vi "Anritsu Power Meter Control Panel (No Objects).vi"(8 "error in (no error)":errorcluster) -> (0 "error out":errorcluster)   [LabVIEW 2009]
doc: "(Dynamic) A user-level application that simulates the physical front panel of the Instrument. Provide the user with buttons to manually control features of the instrument, and provide indicators of its current state."
uses:
  Anritsu Power Meter/Public/Display control.ctl
  Anritsu Power Meter/Public/Range control watts and dBm.ctl
  Anritsu Power Meter/Public/Measuring rate control.ctl
  Anritsu Power Meter/Public/Range Status.ctl
  Anritsu Power Meter/Public/Auto Range control.ctl
  Anritsu Power Meter/Public/Averaging control.ctl
panel:
  in  "VISA Resource Name":refnum<visa-resource-name>="GPIB0::21::INSTR"
  in  "Cluster In":T6={"Averaging"=enum."On", "Units"=enum."Watt", "Measuring rate"=enum."Hold", "Unit Range"=enum."10 mW (+10 dBm)", "Calibration Factor"=-26.67, "Auto Ranging?"=enum."Off"}
  in  "Set Calibration Factor":dbl=-26.67 format="%#5_4g"
  in  "Specify Calibration Factor":bool
  in  "Auto range? 2":bool
  in  "Set Auto Range":T5
  in  "Set Averaging":T1
  out "Averaging":T1
  out "Auto Ranging?":T5
  out "In Range?":T7
  out "Power number":dbl
  out "Power":string
  in  "Set Zero":bool
  in  "Set Unit Range":T4
  in  "Set Measuring Rate":T3
  in  "Specify Range Command":bool
  in  "Set Units":T2
  out "Calibration Factor":dbl
  out "Unit Range":T4
  out "Units":T2
  in  "Query Everything":bool
  in  "Select Measurement Rate":bool
  in  "Averaging?":bool
  in  "Select Unit Display":bool
  in  "Auto range?":bool
  in  "Stop":bool
  in  "Copy actual to set":bool
  in  "Populate fields with member data":bool
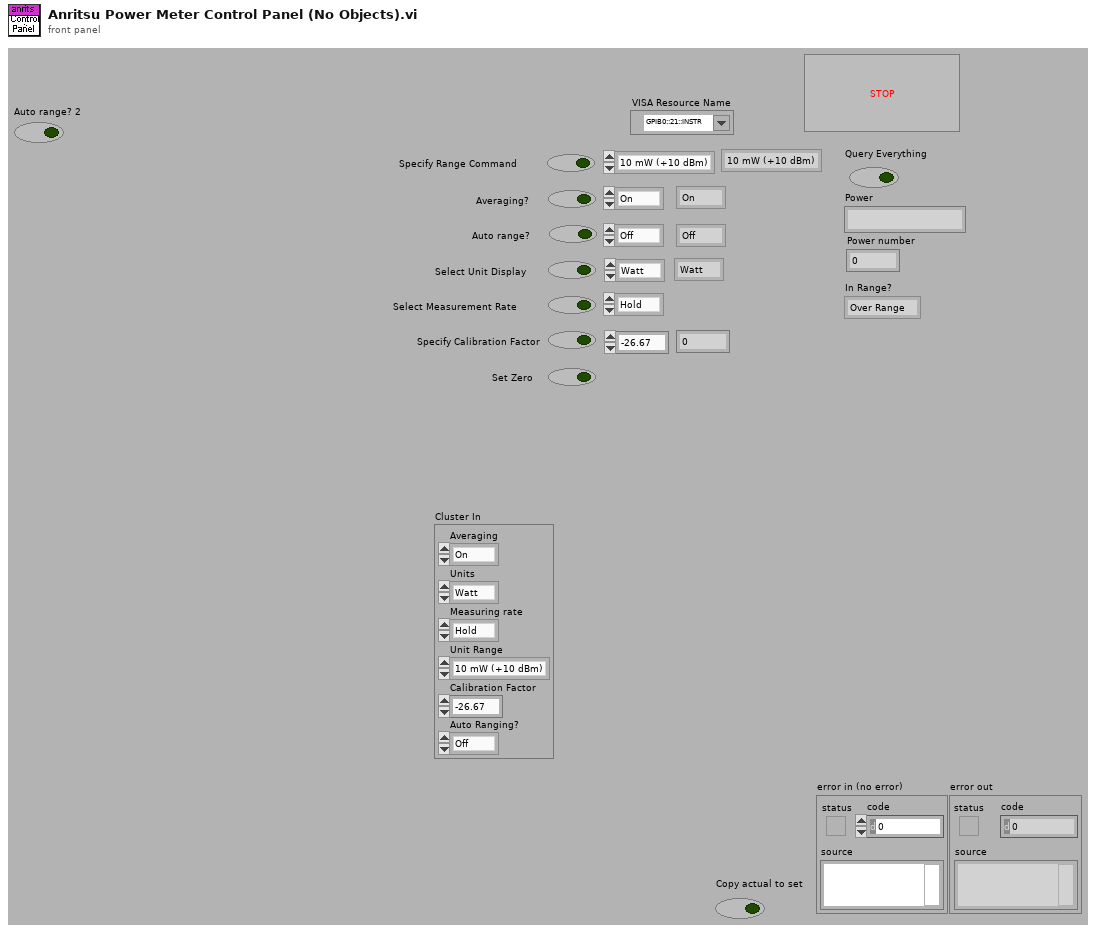
[diagram p1: front panel]
types:
  T1 = typedef "Averaging control.ctl" = enum16{"On", "Off"}
  T2 = typedef "Display control.ctl" = enum16{"Watt", "dBm", "dB (REL)"}
  T3 = typedef "Measuring rate control.ctl" = enum16{"Hold", "Free Run", "Exit Trigger"}
  T4 = typedef "Range control watts and dBm.ctl" = enum16{"10 mW (+10 dBm)", "1 mW (0 dBm)", "100 uW (-10 dBm)", "10 uW (-20 dBm)", "1 uW (-30 dBm)", "100 nW (-40 dBm)", "10 nW (-50 dBm)", "1 nW (-60 dBm)", "100 pW (-70 dBm)", "10 pW (-80 dBm)"}
  T5 = typedef "Auto Range control.ctl" = enum16{"Off", "On"}
  T6 = cluster{"Averaging":T1, "Units":T2, "Measuring rate":T3, "Unit Range":T4, "Calibration Factor":dbl, "Auto Ranging?":T5}
  T7 = typedef "Range Status.ctl" = enum16{"Over Range", "Under Range", "In Range"}
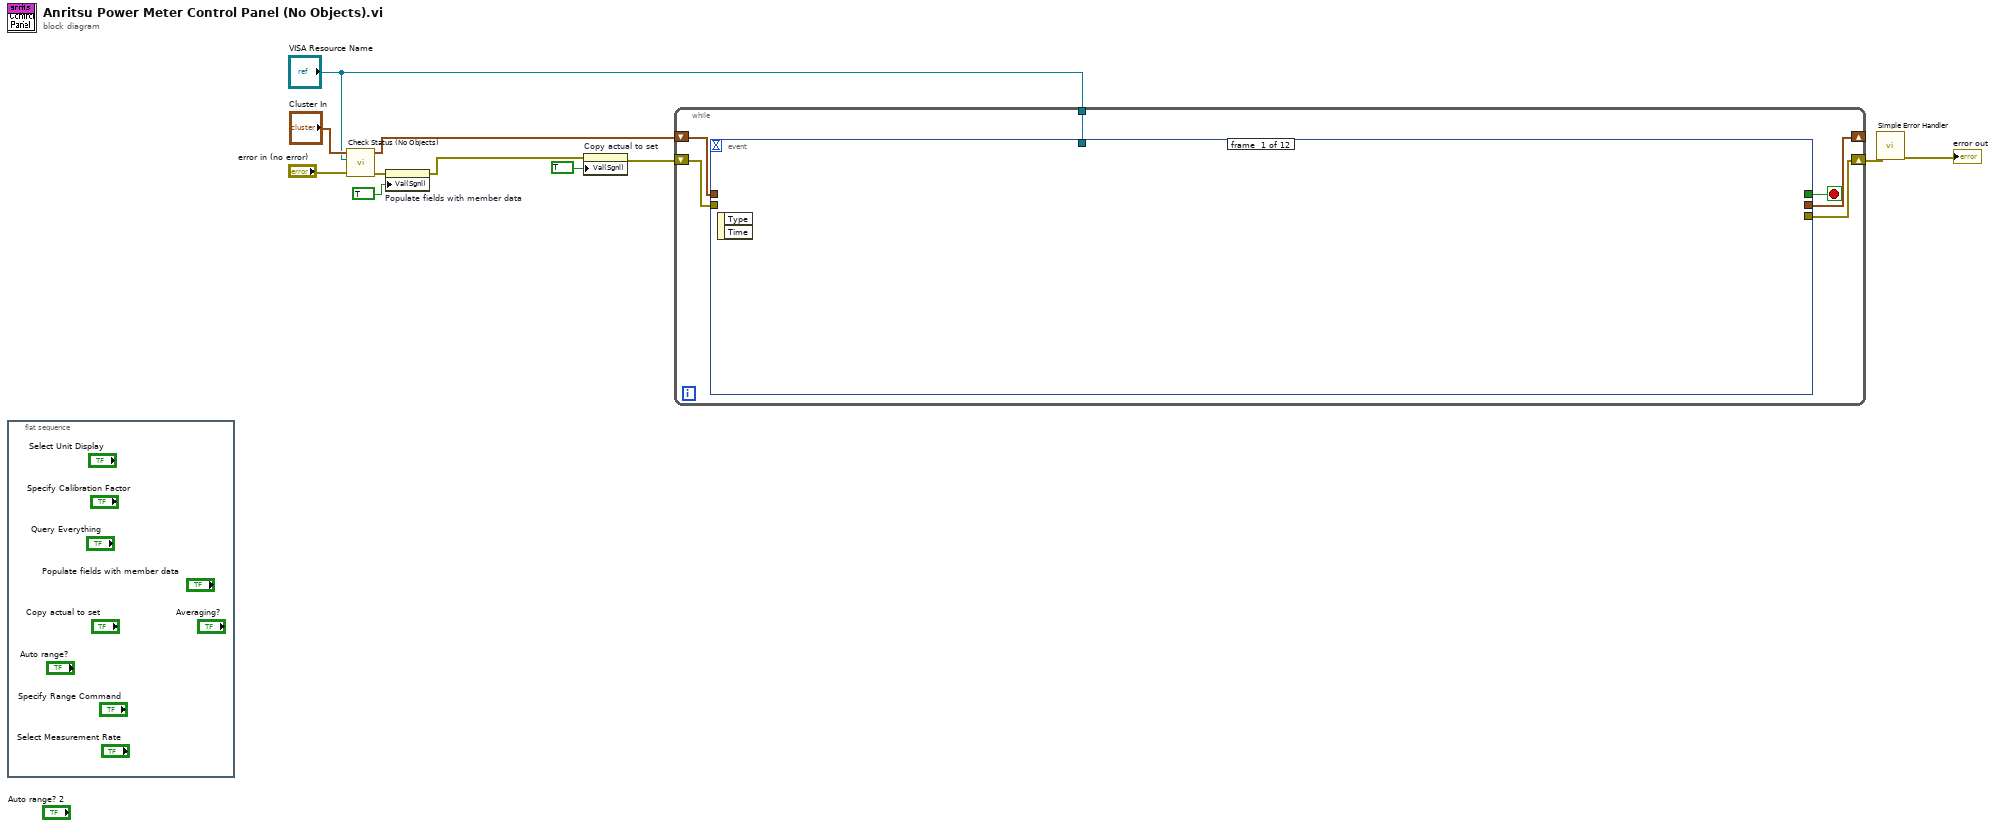
[diagram p0: block diagram]
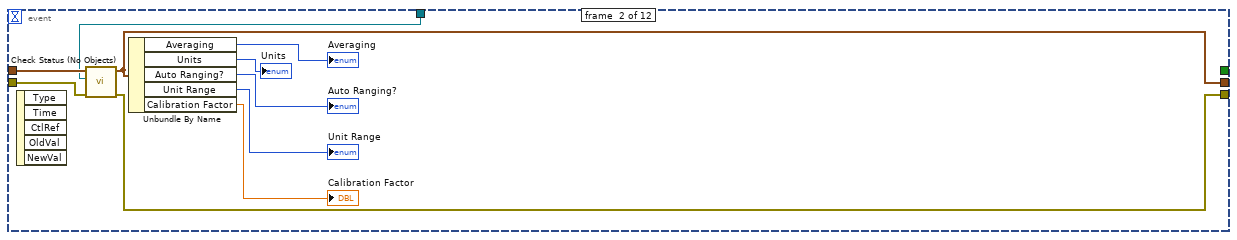
[diagram p2: hidden frame]
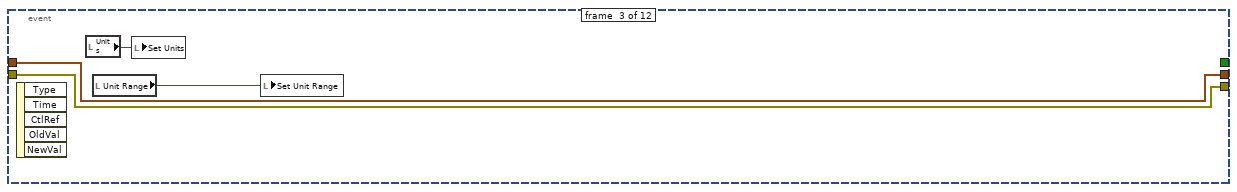
[diagram p3: hidden frame]
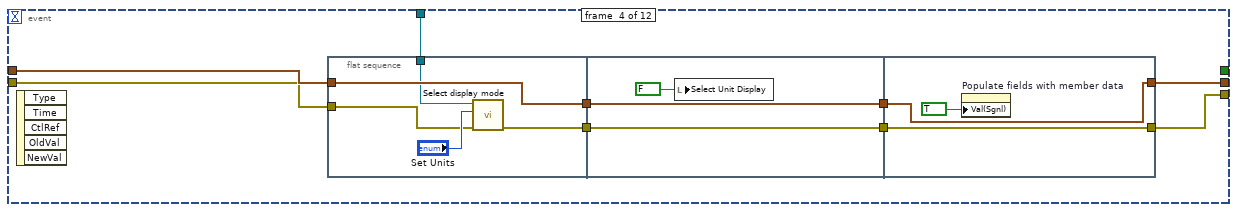
[diagram p4: hidden frame]
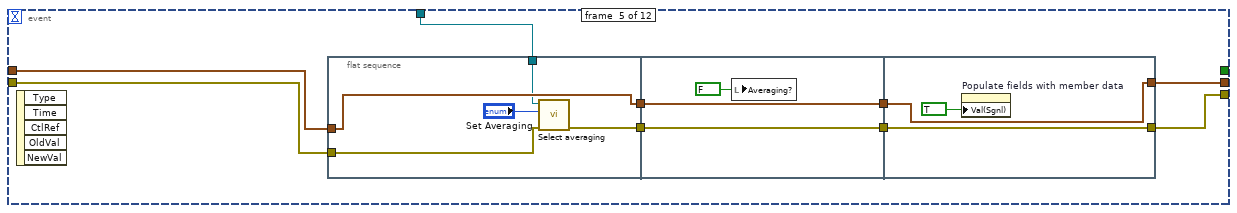
[diagram p5: hidden frame]
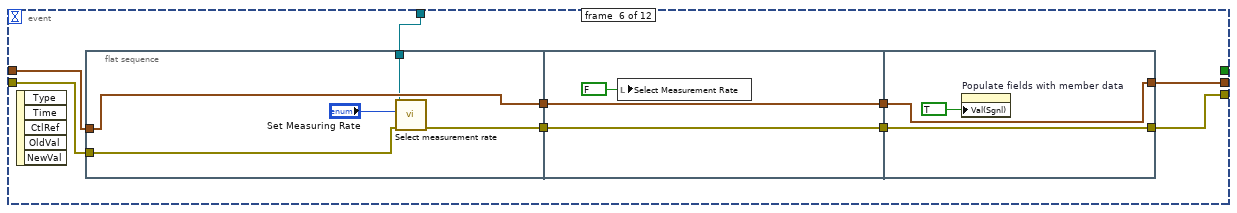
[diagram p6: hidden frame]
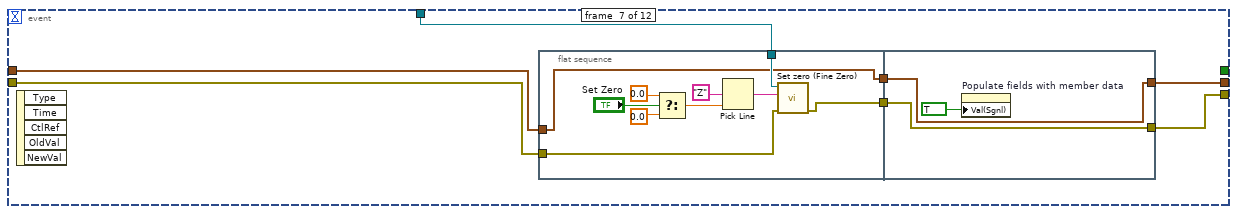
[diagram p7: hidden frame]
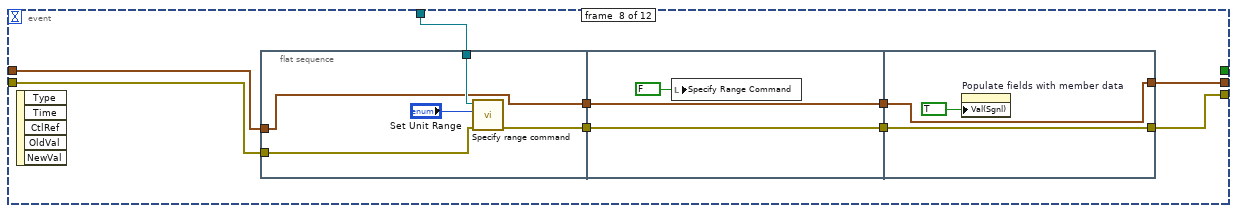
[diagram p8: hidden frame]
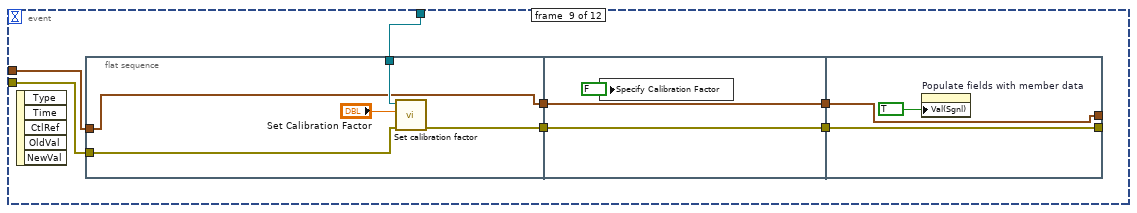
[diagram p9: hidden frame]
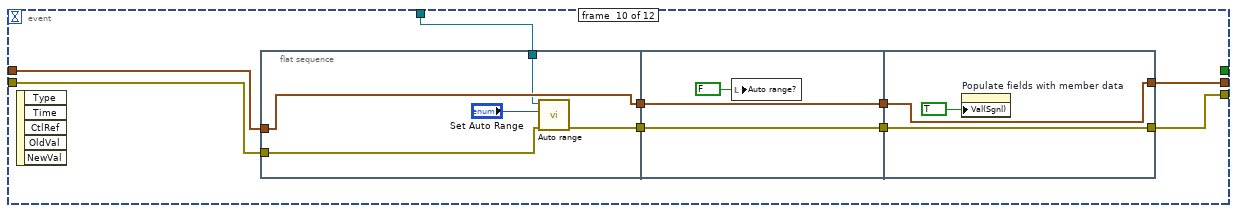
[diagram p10: hidden frame]
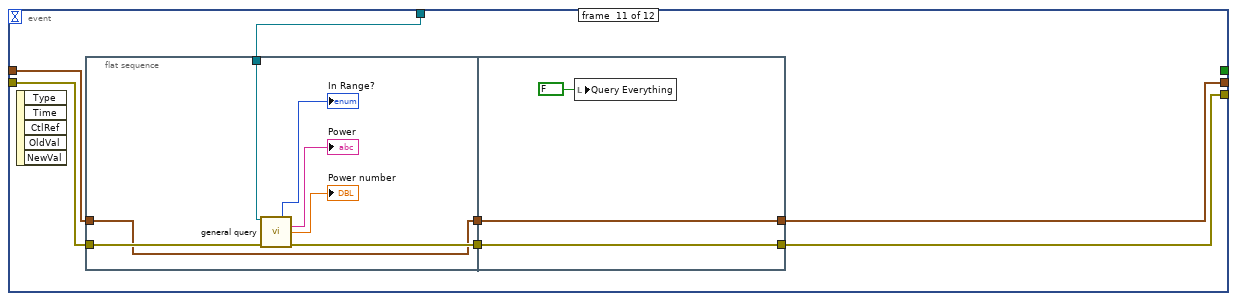
[diagram p11: hidden frame]
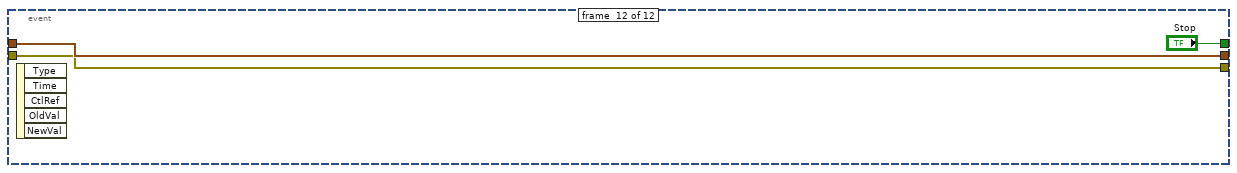
[diagram p12: hidden frame]
diagram:
  n1 = flat-sequence {
    frame #0 {
    }
  }
  n2 = call "Check Status (No Objects).vi"("error in (no error)"="error in (no error)", "VISA Resource Name"="VISA Resource Name", "Cluster In"="Cluster In") -> ("error out"=w10:errorcluster, "Cluster Out"=w8:T6)  [unwired: 5 in, 2 out]
  n3 = property on="Populate fields with member data" class="Bool (strict)"(error in=w10, "Val(Sgnl)"=TRUE ("Value (Signaling)")) -> (error out=w11:errorcluster)  [unwired: 1 in, 1 out]
  n4 = property on="Copy actual to set" class="Bool (strict)"(error in=w11, "Val(Sgnl)"=TRUE ("Value (Signaling)")) -> (error out=w9:errorcluster)  [unwired: 1 in, 1 out]
  n5 = while {
    shift-right: [w15] -> _
    shift-left: w8 -> [w16]
    shift-right: [w14] -> w5
    shift-left: w9 -> [w17]
    tunnel: "VISA Resource Name" -> [w12]
    stop <- w13 stop-if-true
    n6 = event shown="[9] \"Auto range?\": Value Change" {
      selector: _ -> [_ _ _ _ _ _ _ _ _ _ _ _]
      dyn-events: _ -> [_ _ _ _ _ _ _ _ _ _ _ _]
      timeout: _ -> [_ _ _ _ _ _ _ _ _ _ _ _]
      tunnel: w17 -> [_ w23 w28 w39 w59 w79 w97 w117 w133 w157 w176 w188]
      tunnel: w16 -> [_ w24 w29 w40 w60 w80 w98 w118 w134 w158 w175 w189]
      tunnel: [_ w22 w29 w34 w58 w78 w96 w113 _ w156 w172 w189] -> w15
      tunnel: [_ w21 w28 w33 w57 w77 w95 w114 _ w155 w171 w188] -> w14
      tunnel: [_ _ _ _ _ _ _ _ _ _ _ "Stop"] -> w13
      tunnel: w12 -> [_ w18 _ w32 w52 w72 w92 w112 w132 w150 w170 _]
      event #0 {
        n7 = event-data() -> ()  [unwired: 1 in, 2 out]
      }
      event #1 {
        n8 = event-data() -> ()  [unwired: 1 in, 5 out]
        n9 = call "Check Status (No Objects).vi"("error in (no error)"=w23, "VISA Resource Name"=w18, "Cluster In"=w24) -> ("error out"=w21:errorcluster, "Cluster Out"=w22:T6)  [unwired: 5 in, 2 out]
        n10 = Unbundle By Name(w22) -> ("Averaging"=→"Averaging":T1, "Units"=→"Units":T2, "Auto Ranging?"=→"Auto Ranging?":T5, "Unit Range"=→"Unit Range":T4, "Calibration Factor"=→"Calibration Factor":dbl)
      }
      event #2 {
        n11 = event-data() -> ()  [unwired: 1 in, 5 out]
        n12 = local read "Units"() -> (w31:T2)
        n13 = local read "Unit Range"() -> (w30:T4)
        n14 = local write "Set Units"(w31) -> ()
        n15 = local write "Set Unit Range"(w30) -> ()
      }
      event #3 {
        n16 = event-data() -> ()  [unwired: 1 in, 5 out]
        n17 = flat-sequence {
          tunnel: w40 -> [w44]
          tunnel: w39 -> [w43]
          tunnel: [w44] -> w38
          tunnel: [w41] -> w37
          tunnel: w32 -> [w42]
          tunnel: w38 -> [w47]
          tunnel: w37 -> [w46]
          tunnel: [w47] -> w36
          tunnel: [w46] -> w35
          tunnel: w36 -> [w50]
          tunnel: w35 -> [w49]
          tunnel: [w50] -> w34
          tunnel: [w49] -> w33
          frame #0 {
            n18 = call "Select display mode.vi"("error in (no error)"=w43, "Display"="Set Units", "VISA resource name"=w42) -> ("error out"=w41:errorcluster)  [unwired: 7 in, 1 out]
          }
          frame #1 {
            n19 = local write "Select Unit Display"(FALSE) -> ()
          }
          frame #2 {
            n20 = property on="Populate fields with member data" class="Bool (strict)"("Val(Sgnl)"=TRUE ("Value (Signaling)")) -> ()  [unwired: 2 in, 2 out]
          }
        }
      }
      event #4 {
        n21 = event-data() -> ()  [unwired: 1 in, 5 out]
        n22 = flat-sequence {
          tunnel: w60 -> [w63]
          tunnel: w59 -> [w61]
          tunnel: [w63] -> w56
          tunnel: [w64] -> w54
          tunnel: w52 -> [w62]
          tunnel: w56 -> [w68]
          tunnel: [w68] -> w55
          tunnel: w54 -> [w67]
          tunnel: [w67] -> w53
          tunnel: w55 -> [w70]
          tunnel: w53 -> [w69]
          tunnel: [w70] -> w58
          tunnel: [w69] -> w57
          frame #0 {
            n23 = call "Select averaging.vi"("error in (no error)"=w61, "Averaging"="Set Averaging", "VISA resource name"=w62) -> ("error out"=w64:errorcluster)  [unwired: 7 in, 1 out]
          }
          frame #1 {
            n24 = local write "Averaging?"(FALSE) -> ()
          }
          frame #2 {
            n25 = property on="Populate fields with member data" class="Bool (strict)"("Val(Sgnl)"=TRUE ("Value (Signaling)")) -> ()  [unwired: 2 in, 2 out]
          }
        }
      }
      event #5 {
        n26 = event-data() -> ()  [unwired: 1 in, 5 out]
        n27 = flat-sequence {
          tunnel: w80 -> [w83]
          tunnel: w79 -> [w82]
          tunnel: [w83] -> w76
          tunnel: [w84] -> w74
          tunnel: w72 -> [w81]
          tunnel: w76 -> [w88]
          tunnel: [w88] -> w75
          tunnel: w74 -> [w87]
          tunnel: [w87] -> w73
          tunnel: w75 -> [w90]
          tunnel: w73 -> [w89]
          tunnel: [w90] -> w78
          tunnel: [w89] -> w77
          frame #0 {
            n28 = call "Select measurement rate.vi"("error in (no error)"=w82, "Rate"="Set Measuring Rate", "VISA resource name"=w81) -> ("error out"=w84:errorcluster)  [unwired: 7 in, 1 out]
          }
          frame #1 {
            n29 = local write "Select Measurement Rate"(FALSE) -> ()
          }
          frame #2 {
            n30 = property on="Populate fields with member data" class="Bool (strict)"("Val(Sgnl)"=TRUE ("Value (Signaling)")) -> ()  [unwired: 2 in, 2 out]
          }
        }
      }
      event #6 {
        n31 = event-data() -> ()  [unwired: 1 in, 5 out]
        n32 = flat-sequence {
          tunnel: w97 -> [w100]
          tunnel: w98 -> [w99]
          tunnel: [w99] -> w94
          tunnel: [w102] -> w93
          tunnel: w92 -> [w101]
          tunnel: w94 -> [w110]
          tunnel: w93 -> [w109]
          tunnel: [w110] -> w96
          tunnel: [w109] -> w95
          frame #0 {
            n33 = Select(t=0.0, s="Set Zero", f=0.0) -> (s? t:f=w106:dbl)
            n34 = Pick Line(multi-line string="Z", line index=w106) -> (output string=w104:string)  [unwired: 1 in]
            n35 = call "Set zero (Fine Zero).vi"("error in (no error)"=w100, "Code"=w104, "VISA resource name"=w101) -> ("error out"=w102:errorcluster)  [unwired: 7 in, 1 out]
          }
          frame #1 {
            n36 = property on="Populate fields with member data" class="Bool (strict)"("Val(Sgnl)"=TRUE ("Value (Signaling)")) -> ()  [unwired: 2 in, 2 out]
          }
        }
      }
      event #7 {
        n37 = event-data() -> ()  [unwired: 1 in, 5 out]
        n38 = flat-sequence {
          tunnel: [w123] -> w120
          tunnel: [w122] -> w119
          tunnel: w118 -> [w123]
          tunnel: w117 -> [w121]
          tunnel: w112 -> [w124]
          tunnel: w120 -> [w127]
          tunnel: w119 -> [w126]
          tunnel: [w127] -> w116
          tunnel: [w126] -> w115
          tunnel: w116 -> [w130]
          tunnel: w115 -> [w129]
          tunnel: [w130] -> w113
          tunnel: [w129] -> w114
          frame #0 {
            n39 = call "Specify range command.vi"("error in (no error)"=w121, "Range"="Set Unit Range", "VISA resource name"=w124) -> ("error out"=w122:errorcluster)  [unwired: 7 in, 1 out]
          }
          frame #1 {
            n40 = local write "Specify Range Command"(FALSE) -> ()
          }
          frame #2 {
            n41 = property on="Populate fields with member data" class="Bool (strict)"("Val(Sgnl)"=TRUE ("Value (Signaling)")) -> ()  [unwired: 2 in, 2 out]
          }
        }
      }
      event #8 {
        n42 = event-data() -> ()  [unwired: 1 in, 5 out]
        n43 = flat-sequence {
          tunnel: [w139] -> w138
          tunnel: [w142] -> w137
          tunnel: w134 -> [w139]
          tunnel: w133 -> [w140]
          tunnel: w132 -> [w141]
          tunnel: w138 -> [w146]
          tunnel: [w146] -> w136
          tunnel: w137 -> [w145]
          tunnel: [w145] -> w135
          tunnel: w136 -> [w149]
          tunnel: w135 -> [w148]
          tunnel: [w149] -> _
          tunnel: [w148] -> _
          frame #0 {
            n44 = call "Set calibration factor.vi"("error in (no error)"=w140, "Calibration Factor"="Set Calibration Factor", "VISA resource name"=w141) -> ("error out"=w142:errorcluster)  [unwired: 7 in, 1 out]
          }
          frame #1 {
            n45 = local write "Specify Calibration Factor"(FALSE) -> ()
          }
          frame #2 {
            n46 = property on="Populate fields with member data" class="Bool (strict)"("Val(Sgnl)"=TRUE ("Value (Signaling)")) -> ()  [unwired: 2 in, 2 out]
          }
        }
      }
      event #9 {
        n47 = event-data() -> ()  [unwired: 1 in, 5 out]
        n48 = flat-sequence {
          tunnel: [w162] -> w153
          tunnel: w158 -> [w161]
          tunnel: w157 -> [w159]
          tunnel: [w161] -> w151
          tunnel: w150 -> [w160]
          tunnel: [w166] -> w154
          tunnel: w153 -> [w165]
          tunnel: [w165] -> w152
          tunnel: w151 -> [w166]
          tunnel: w154 -> [w169]
          tunnel: w152 -> [w168]
          tunnel: [w169] -> w156
          tunnel: [w168] -> w155
          frame #0 {
            n49 = call "Auto range.vi"("error in (no error)"=w159, "Auto Ranging?"="Set Auto Range", "VISA resource name"=w160) -> ("error out"=w162:errorcluster)  [unwired: 7 in, 1 out]
          }
          frame #1 {
            n50 = local write "Auto range?"(FALSE) -> ()
          }
          frame #2 {
            n51 = property on="Populate fields with member data" class="Bool (strict)"("Val(Sgnl)"=TRUE ("Value (Signaling)")) -> ()  [unwired: 2 in, 2 out]
          }
        }
      }
      event #10 {
        n52 = event-data() -> ()  [unwired: 1 in, 5 out]
        n53 = flat-sequence {
          tunnel: w176 -> [w178]
          tunnel: w175 -> [w177]
          tunnel: [w180] -> w174
          tunnel: [w177] -> w173
          tunnel: w170 -> [w179]
          tunnel: w174 -> [w184]
          tunnel: w173 -> [w185]
          tunnel: [w185] -> w172
          tunnel: [w184] -> w171
          frame #0 {
            n54 = call "general query.vi"("VISA resource name"=w179, "error in (no error)"=w178) -> ("In Range?"=→"In Range?":T7, "Power"=→"Power":string, "Power num"=→"Power number":dbl, "error out"=w180:errorcluster)  [unwired: 5 in, 5 out]
          }
          frame #1 {
            n55 = local write "Query Everything"(FALSE ("Value (Signaling)")) -> ()
          }
        }
      }
      event #11 {
        n56 = event-data() -> ()  [unwired: 1 in, 5 out]
      }
    }
  }
  n57 = call <vilib>:"Simple Error Handler.vi"("error in (no error)"=w5) -> ("error out"=→"error out":errorcluster)  [unwired: 1 in, 7 out]
